vi "AutoTurnGyro.vi"(7 "Sensor (Gyro)":enum16{"Gyro", "Vision", "Encoder"}(ring), 8 "error in":errorcluster, 10 "Turn Amount":i32=45, 11 "Initial Angle":dbl) -> (0 "error out":errorcluster, 3 "Target Angle Out":dbl)   [LabVIEW 2012]
doc: "This VI is called when autonomous begins, and will automatically be terminated when autonomous ends. You can carry out timed or sensor driven robot movement independently without needing to return to the caller."
uses:
  <vilib>/Rock Robotics/WPI/RobotDrive/WPI_RobotDriveGetSetRefNum.vi
  Robot Global Data.vi
panel:
  out "Loop (Hz)":dbl
  out "Output":dbl
  in  "PID gains":T1={"proportional gain (Kc)"=0.025, "integral time (Ti, min)"=0.0, "derivative time (Td, min)"=0.0} {"proportional gain (Kc)" format="%_6f"; "integral time (Ti, min)" format="%_6f"; "derivative time (Td, min)" format="%_6f"}
  out "Graph":cluster{dbl, dbl, "Time for happy (ms)":dbl}(graph)
  out "PID Output":dbl format="%.2f"
  out "Error":dbl
  out "Current Angle":dbl
  # "Low gear\nMax turn - 0.71\nMin turn - 0.45"
  # "Curve Value Input Not used when using Gyro"
  # "\"-\" Turns Left\n\"+\" Turns Right"
  # "If Using Gyro:\nEnter Turn amount in Degrees:\n\"-\" AngleTurns Left\n\"+\" Angle Turns Right"
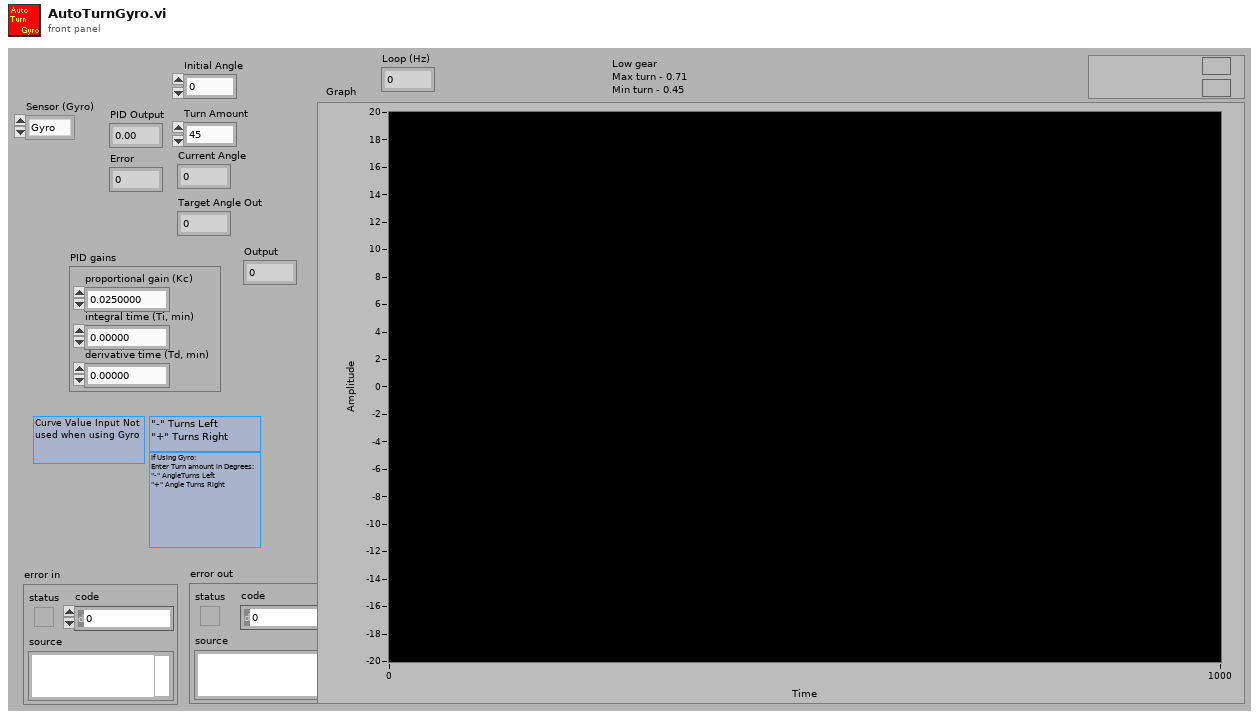
[diagram p1: front panel]
types:
  T1 = cluster{"proportional gain (Kc)":dbl, "integral time (Ti, min)":dbl, "derivative time (Td, min)":dbl}
  T2 = typedef "WPI_RobotDriveDevRef.ctl" = cluster{"DevStatus":errorcluster, "Motors[]":T3[], "Square Inputs":bool, "Max Output":dbl, "Isochronous":bool}
  T3 = typedef "WPI_MotorControlDeviceRef.ctl" = cluster{"DeviceStatus":errorcluster, "Type":enum16{"PWM", "CAN"}, "PWM":cluster{"Digital Module":T4, "PWM Channel":T5, "DeadBand":T6}, "CAN":cluster{"Device Number":u8, "Control Mode":T7, "Semaphore":T8, "Max Vout":dbl}, "Invert":bool, "TransformRef":T9, "InvTransformRef":T9}
  T4 = typedef "FPGA_TypedefDigitalModule.ctl" = enum16{"Digital Module 1", "Digital Module 2"}
  T5 = typedef "FPGA_DIOPWMChannel.ctl" = enum8{"PWM 1", "PWM 2", "PWM 3", "PWM 4", "PWM 5", "PWM 6", "PWM 7", "PWM 8", "PWM 9", "PWM 10", "Invalid"}
  T6 = typedef "WPI_PWMDeadband.ctl" = cluster{"Name":string, "maxPositivePwm":i32, "minPositivePwm":i32, "centerPwm":i32, "maxNegativePwm":i32, "minNegativePwm":i32, "angularRange":u16}
  T7 = typedef "WPI_CANJaguar_ControlMode.ctl" = enum8{"Percent VBus", "Current", "Speed", "Position", "Voltage"}
  T8 = typedef "Semaphore RefNum" = refnum<k1>
  T9 = typedef "WPI_PWMTransform_ConPane.ctl" = refnum<vi>
  T10 = typedef "WPI_GyroDevRef.ctl" = cluster{"DevStatus":errorcluster, "Analog Module":T11, "Analog Channel":T12, "Offset":dbl, "Gain (VoltsPerDegree/Second)":dbl}
  T11 = typedef "FPGA_TypedefAnalogModule.ctl" = enum16{"Analog Module 1", "Analog Module 2"}
  T12 = typedef "FPGA_AIChannel.ctl" = enum8{"AI 1", "AI 2", "AI 3", "AI 4", "AI 5", "AI 6", "AI 7", "AI 8", "Invalid"}
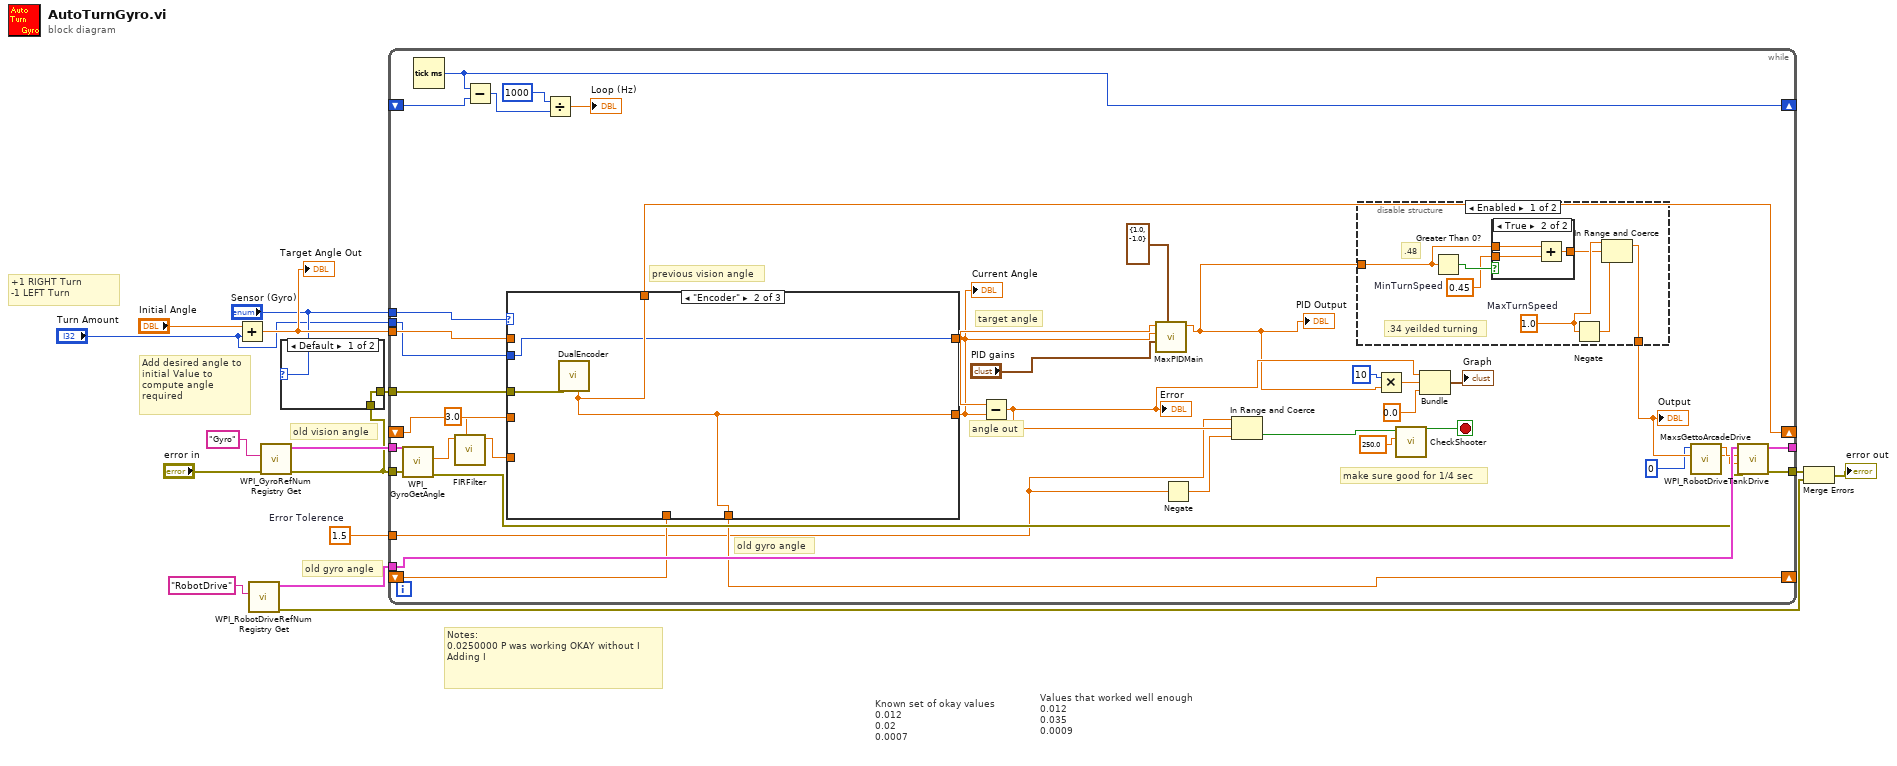
[diagram p0: block diagram]
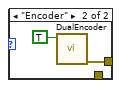
[diagram p2: hidden frame]
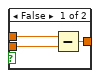
[diagram p3: hidden frame]
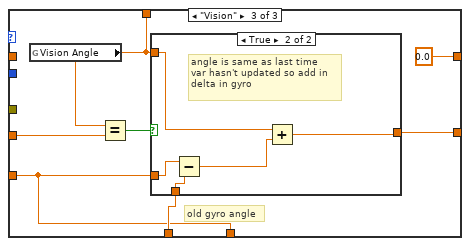
[diagram p6: hidden frame]
diagram:
  w12 = 1.5  # Error Tolerence
  # "Values that worked well enough\n0.012\n0.035\n0.0009"
  # "Known set of okay values\n0.012\n0.02\n0.0007"
  # "Notes:\n0.0250000 P was working OKAY without I\nAdding I"
  # "old vision angle"
  # "old gyro angle"
  # "+1 RIGHT Turn\n-1 LEFT Turn"
  # "Add desired angle to initial Value to\ncompute angle required"
  n1 = Add(x="Initial Angle", y="Turn Amount") -> (x+y=w7:dbl)
  "Target Angle Out" <- w7
  n2 = call <vilib>:"WPI_RobotDriveRefNum Registry Get.vi"("refnum name"="RobotDrive") -> ("error out"=w8:errorcluster, "RobotDriveDevRef"=w10:T2)  [unwired: 9 in]
  n3 = call <vilib>:"WPI_GyroRefNum Registry Get.vi"("error in (no error)"="error in", "refnum name"="Gyro") -> ("error out"=w2:errorcluster, "GyroDevRef"=w11:T10)  [unwired: 8 in]
  n4 = case shown="Default" "Sensor (Gyro)" {
    tunnel: [w16 w18] -> w3
    tunnel: w2 -> [w16 _]
    frame Default {
    }
    frame "Encoder" {
      n5 = call "DualEncoder.vi"("Reset?"=TRUE) -> ("error out"=w18:errorcluster)  [unwired: 6 in, 4 out]
    }
  }
  n6 = while {
    tunnel: [w59] -> _
    tunnel: [w58] -> w9
    tunnel: "Sensor (Gyro)" -> [w56]
    tunnel: w12 -> [w20]
    tunnel: w11 -> [w46]
    tunnel: w2 -> [w45]
    tunnel: w10 -> [w53]
    tunnel: w7 -> [w52]
    shift-right: [w41] -> _
    shift-left: _ -> [w47]
    shift-right: [w43] -> _
    shift-left: _ -> [w42]
    shift-right: [w29] -> _
    shift-left: _ -> [w28]
    tunnel: w3 -> [w21]
    tunnel: "Turn Amount" -> [w19]
    stop <- w40 stop-if-true
    # "old gyro angle"
    # "target angle"
    # "angle out"
    # "previous vision angle"
    # "make sure good for 1/4 sec"
    n7 = call <vilib>:"WPI_GyroGetAngle.vi"("error in (no error)"=w45, "GyroDevRef"=w46) -> ("error out"=w44:errorcluster, "Angle"=w23:dbl)  [unwired: 8 out]
    n8 = Tick Count (ms)() -> (millisecond timer value=w29:u32)
    n9 = call "FIRFilter.vi"("Filter Size"=3.0, "Input"=w23) -> ("Output"=w24:dbl)  [unwired: 9 in]
    n10 = Subtract(x=w29, y=w28) -> (x-y=w27:u32)
    n11 = case shown="\"Encoder\"" w56 {
      tunnel: [w74 w77 w84] -> w48
      tunnel: w52 -> [w75 _ _]
      tunnel: [w75 w76 0.0] -> w51
      tunnel: w47 -> [_ _ w79]
      tunnel: w24 -> [w74 _ w81]
      tunnel: [w74 w77 w81] -> w43
      tunnel: w42 -> [_ _ w82]
      tunnel: [w74 w77 w80] -> w41
      tunnel: w21 -> [_ w78 _]
      tunnel: w19 -> [_ w76 _]
      frame "Gyro", Default {
        # "is using gyro to turn feed through gyro angle"
      }
      frame "Encoder" {
        n12 = call "DualEncoder.vi"("error in (no error)"=w78) -> ("Angle (degrees)"=w77:dbl)  [unwired: 6 in, 4 out]
      }
      frame "Vision" {
        # "old gyro angle"
        n13 = global read "Robot Global Data.vi" "Vision Angle"() -> (w80:dbl)
        n14 = Equal?(x=w80, y=w79) -> (x = y?=w83:bool)
        n15 = case shown="True" w83 {
          tunnel: [w86 w87] -> w84
          tunnel: w80 -> [w86 w89]
          tunnel: w82 -> [_ w90]
          tunnel: w81 -> [_ w91]
          frame False {
            # "if vision angle isn't the same\nas last time. this means it updated\nand is good to use"
          }
          frame True {
            # "angle is same as last time\nvar hasn't updated so add in\ndelta in gyro"
            n16 = Subtract(x=w91, y=w90) -> (x-y=w88:dbl)
            n17 = Add(x=w89, y=w88) -> (x+y=w87:dbl)
          }
        }
      }
    }
    "Current Angle" <- w48
    n18 = Divide(x=1000, y=w27) -> (x/y=→"Loop (Hz)":dbl)
    n19 = Subtract(x=w51, y=w48) -> (x-y=w55:dbl)
    "Error" <- w55
    n20 = call "MaxPIDMain.vi"("Output Range"=cluster{"output high":dbl, "output low":dbl} {"output high"=1.0, "output low"=-1.0} ("output range"), "PID gains"="PID gains", "process variable"=w48, "setpoint"=w51) -> ("Output"=w34:dbl)  [unwired: 6 in, 1 out]
    "PID Output" <- w34
    n21 = Negate(x=w20) -> (-x=w54:dbl)
    n22 = In Range and Coerce(upper limit=w20, x=w55, lower limit=w54) -> (In Range?=w39:bool)  [unwired: 1 out]
    n23 = disable-structure shown="Enabled" {
      disable-tunnel: [w66 w73] -> w31
      disable-tunnel: w34 -> [w60 w73]
      frame Enabled {
        w64 = 1.0  # MaxTurnSpeed
        w61 = 0.45  # MinTurnSpeed
        # ".48"
        # ".34 yeilded turning"
        n24 = Greater Than 0?(x=w60) -> (x > 0?=w62:bool)
        n25 = case shown="True" w62 {
          tunnel: [w68 w72] -> w63
          tunnel: w60 -> [w69 w71]
          tunnel: w61 -> [w67 w70]
          frame False {
            n26 = Subtract(x=w69, y=w67) -> (x-y=w68:dbl)
          }
          frame True {
            n27 = Add(x=w71, y=w70) -> (x+y=w72:dbl)
          }
        }
        n28 = Negate(x=w64) -> (-x=w65:dbl)
        n29 = In Range and Coerce(upper limit=w64, x=w63, lower limit=w65) -> (coerced(x)=w66:dbl)  [unwired: 1 out]
      }
      frame Disabled {
      }
    }
    "Output" <- w31
    n30 = Multiply(x=10, y=w34) -> (x*y=w50:dbl)
    n31 = call "CheckShooter.vi"("Time for happy (ms)"=250.0, "Shooter Good?"=w39) -> ("Good to shoot"=w40:bool)  [unwired: 9 in]
    n32 = Bundle(w55, w50, "Time for happy (ms)"=0.0) -> (→"Graph":cluster{dbl, dbl, "Time for happy (ms)":dbl})  [unwired: 1 out]
    n33 = call "MaxsGettoArcadeDrive.vi"("Driver X In"=w31, "Driver Y In"=0) -> ("Right Out"=w32:dbl, "Left Out"=w33:dbl)  [unwired: 8 in]
    n34 = call <vilib>:"WPI_RobotDriveTankDrive.vi"("error in (no error)"=w44, "Right axis value"=w32, "Left axis value"=w33, "RobotDriveDevRef"=w53) -> ("error out"=w58:errorcluster, "RobotDriveDevRef"=w59:T2)  [unwired: 5 in, 1 out]
  }
  n35 = Merge Errors(w9, w8) -> (→"error out":errorcluster)
